vi "usrp_init (SubVI).vi"(10 "IQ Rate [S/sec]":dbl=1000000.0 format="%#_6p") -> (0 "error out":errorcluster, 1 "IVI Refnum out":refnum<k15>, 3 "Enabled Channel out":string(combo)="0")   [LabVIEW 2017]
panel:
  in  "Enabled Channel in":string(combo)="0"
  in  "IVI Refnum in":refnum<k15>="192.168.10.2"
  in  "Active Antenna":string="RX1"
  out "Coerced Gain":dbl=1.0 format="%#_6f"
  out "Coerced Carrier Frequency":dbl format="%#_6p"
  out "Coerced IQ Rate [S/sec]":dbl=1000000.0 format="%#_6p"
  in  "Gain":dbl=1.0 format="%#_6f"
  in  "Carrier Frequency":dbl format="%#_6p"
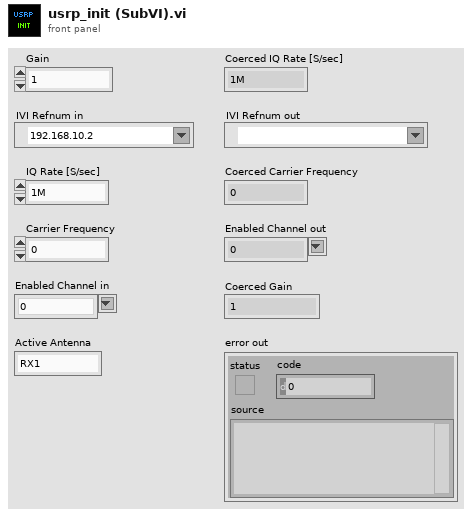
[diagram p1: front panel]
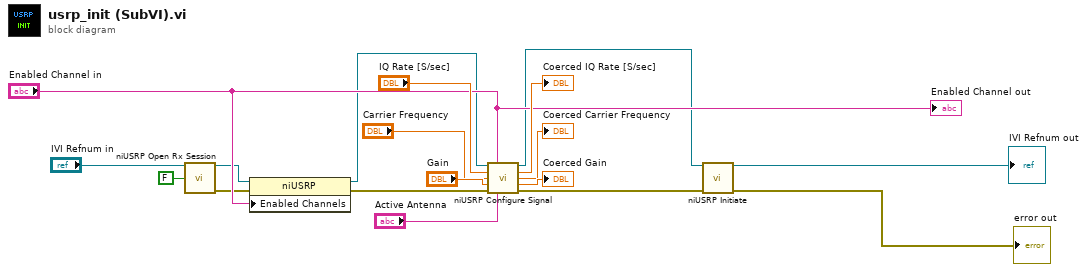
[diagram p0: block diagram]
diagram:
  n1 = call <instrlib>:"niUSRP Open Rx Session.vi"("device names"="IVI Refnum in", "reset"=FALSE) -> ("session handle out"=w9:refnum<k15>, "error out"=w11:errorcluster)  [unwired: 12 in]
  n2 = property class="niUSRP"(reference=w9, error in=w11, "Enabled Channels"="Enabled Channel in") -> (reference out=w10:refnum<k15>, error out=w12:errorcluster)
  n3 = call <instrlib>:"niUSRP Configure Signal.vi"("session handle"=w10, "channel list"="Enabled Channel in", "IQ rate"="IQ Rate [S/sec]", "carrier frequency"="Carrier Frequency", "gain"="Gain", "error in (no error)"=w12, "active antenna"="Active Antenna") -> ("session handle out"=w7:refnum<k15>, "coerced IQ rate"=→"Coerced IQ Rate [S/sec]":dbl, "coerced carrier frequency"=→"Coerced Carrier Frequency":dbl, "coerced gain"=→"Coerced Gain":dbl, "error out"=w8:errorcluster)  [unwired: 4 in]
  n4 = call <instrlib>:"niUSRP Initiate.vi"("session handle"=w7, "error in (no error)"=w8) -> ("session handle out"=→"IVI Refnum out":refnum<k15>, "error out"=→"error out":errorcluster)  [unwired: 12 in]
  "Enabled Channel out" <- "Enabled Channel in"
